vi "Serialize - Text.vi"(8 "error in":errorcluster, 11 "Heater Data in":refnum<class "Heater Data.lvclass">) -> (0 "error out":errorcluster, 2 "Serialized Text":string, 3 "Heater Data out":refnum<class "Heater Data.lvclass">)   [LabVIEW 2017, in "Controller.lvlib" / "Heater Data.lvclass"]
uses:
  Heater Data.lvclass
  Heater Data.lvclass/Heater Data.ctl
  <vilib>/MSR Consulting, LLC/General Reuse/Data/Data.lvclass
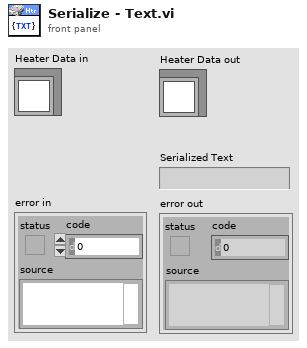
[diagram p1: front panel]
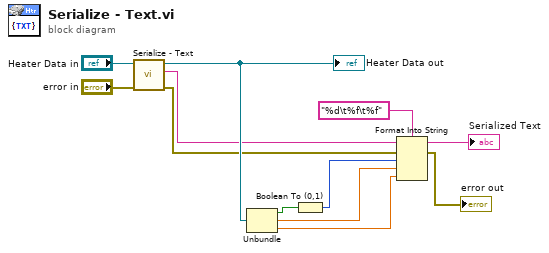
[diagram p0: block diagram]
diagram:
  n1 = call-parent "Serialize - Text.vi"("error in"="error in", "Data in"="Heater Data in") -> ("error out"=w1:errorcluster, "Serialized Text"=w9:string, "Data out"=w10:refnum<class "Heater Data.lvclass">)  [unwired: 7 in]
  "Heater Data out" <- w10
  n2 = Unbundle(w10) -> (w7:bool, w5:dbl, w4:dbl)
  n3 = Boolean To (0,1)(Boolean=w7) -> (0, 1=w6:i16)
  n4 = Format Into String(format string="%d\t%f\t%f", initial string=w9, error in=w1, w6, w5, w4) -> (resulting string=→"Serialized Text":string, error out=→"error out":errorcluster)
